vi "read_data_with_UDP.vi"(8 "error_in":errorcluster, 11 "udp_ref_in":refnum<k16>) -> (0 "error_out":errorcluster, 2 "data_out":dbl[](array[numeric]), 3 "udp_ref_out":refnum<k16>)   [LabVIEW 2020]
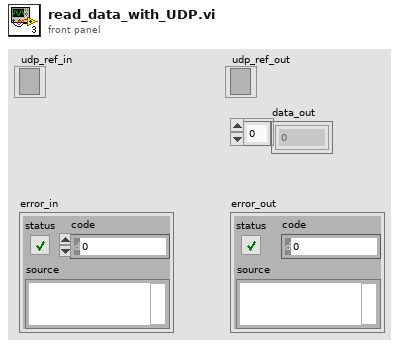
[diagram p1: front panel]
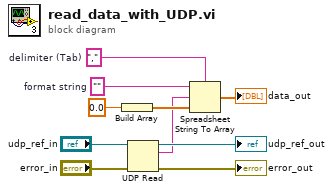
[diagram p0: block diagram]
diagram:
  w8 = ","  # delimiter (Tab)
  w7 = ""  # format string
  n1 = Build Array(0.0) -> (w6:dbl[])
  n2 = UDP Read(connection ID="udp_ref_in", 8:"error_in") -> (data out=w1:string, error out=→"error_out":errorcluster, 3:→"udp_ref_out":refnum<k16>)  [unwired: 2 in, 2 out]
  n3 = Spreadsheet String To Array(delimiter (Tab)=w8, format string=w7, spreadsheet string=w1, array type (2D Dbl)=w6) -> (array=→"data_out":dbl[])
